vi "Clear MDIF file.vi"(8 "error in (no error)":errorcluster, 11 "MDIF reference in":refnum<k24>) -> (0 "error out":errorcluster, 3 "MDIF reference out":refnum<k24>)   [LabVIEW 2023, in "NI_HFNetworkAnalysis.lvlib"]
doc: "Clear all MDIF blocks in memory for the referenced MDIF file.\n\n<b>Notes</b>\n- Only the MDIF blocks in memory are cleared.\n- In order to clear the content of the referenced MDIF file on disk as well, use <b>Save MDIF File.vi</b> after this VI."
uses:
  NI_HFNetworkAnalysis.lvlib
  C:/srd-semi-rfcal-software/AuxTools/STSRFFixtureCharactUtility/Source/Code Modules/Fixture/Dependencies/HFNetworkAnalysis/Support Files/NACE.Utils.Data.dll
  Support Files/NACE.Utils.Data.dll
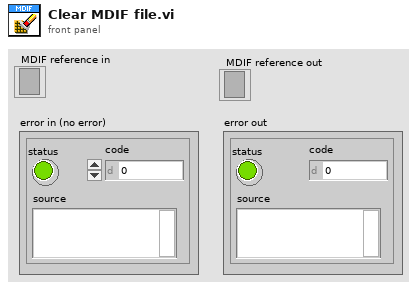
[diagram p1: front panel]
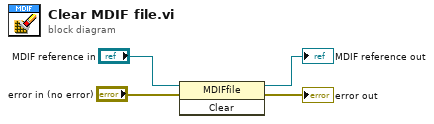
[diagram p0: block diagram]
diagram:
  n1 = invoke class="MDIFfile" method="Clear"(reference="MDIF reference in", error in="error in (no error)") -> (reference out=→"MDIF reference out":refnum<k24>, error out=→"error out":errorcluster)  [unwired: 1 in, 1 out]
